vi "Compare Values.vi"(10 "P2":dbl, 11 "P1":dbl) -> (3 "Abs Diff":dbl)   [LabVIEW 2015]
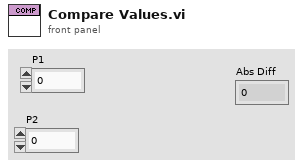
[diagram p1: front panel]
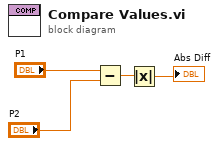
[diagram p0: block diagram]
diagram:
  n1 = Subtract(x="P1", y="P2") -> (x-y=w2:dbl)
  n2 = Absolute Value(x=w2) -> (abs(x)=→"Abs Diff":dbl)
